vi "Trainging_Program_redesign_1세부통합.vi"() -> ()   [LabVIEW 2014]
uses:
  <vilib>/DAQmx/create/channels.llb/DAQmx Create Channel (AI-Voltage-Basic).vi
  <vilib>/DAQmx/configure/timing.llb/DAQmx Timing (Sample Clock).vi
  <vilib>/DAQmx/read.llb/DAQmx Read (Analog 1D Wfm NChan NSamp).vi
  <vilib>/Utility/file.llb/Write To Spreadsheet File (I64).vi
  <vilib>/Utility/file.llb/Write To Spreadsheet File (DBL).vi
  NeuroSky_Dll_Call/Debug/NeuroSky_Dll_Call.dll
panel:
  out "큐사인":bool
  out "실험종료":bool=TRUE
  out "icon_온도":bool
  out "icon_자판":bool
  out "icon_침대":bool
  out "icon_기계":bool
  out "icon_응급":bool=TRUE
  out "icon_용변":bool
  out "error out":errorcluster={"status"=TRUE, "code"=10, "source"="Create Folder in Trainging_Set_For_ LDA_Matrix_RSVP.vi<APPEND>\nC:\\Emotion_Research\\_Training_Test(LDA)\\2014-08-30"}
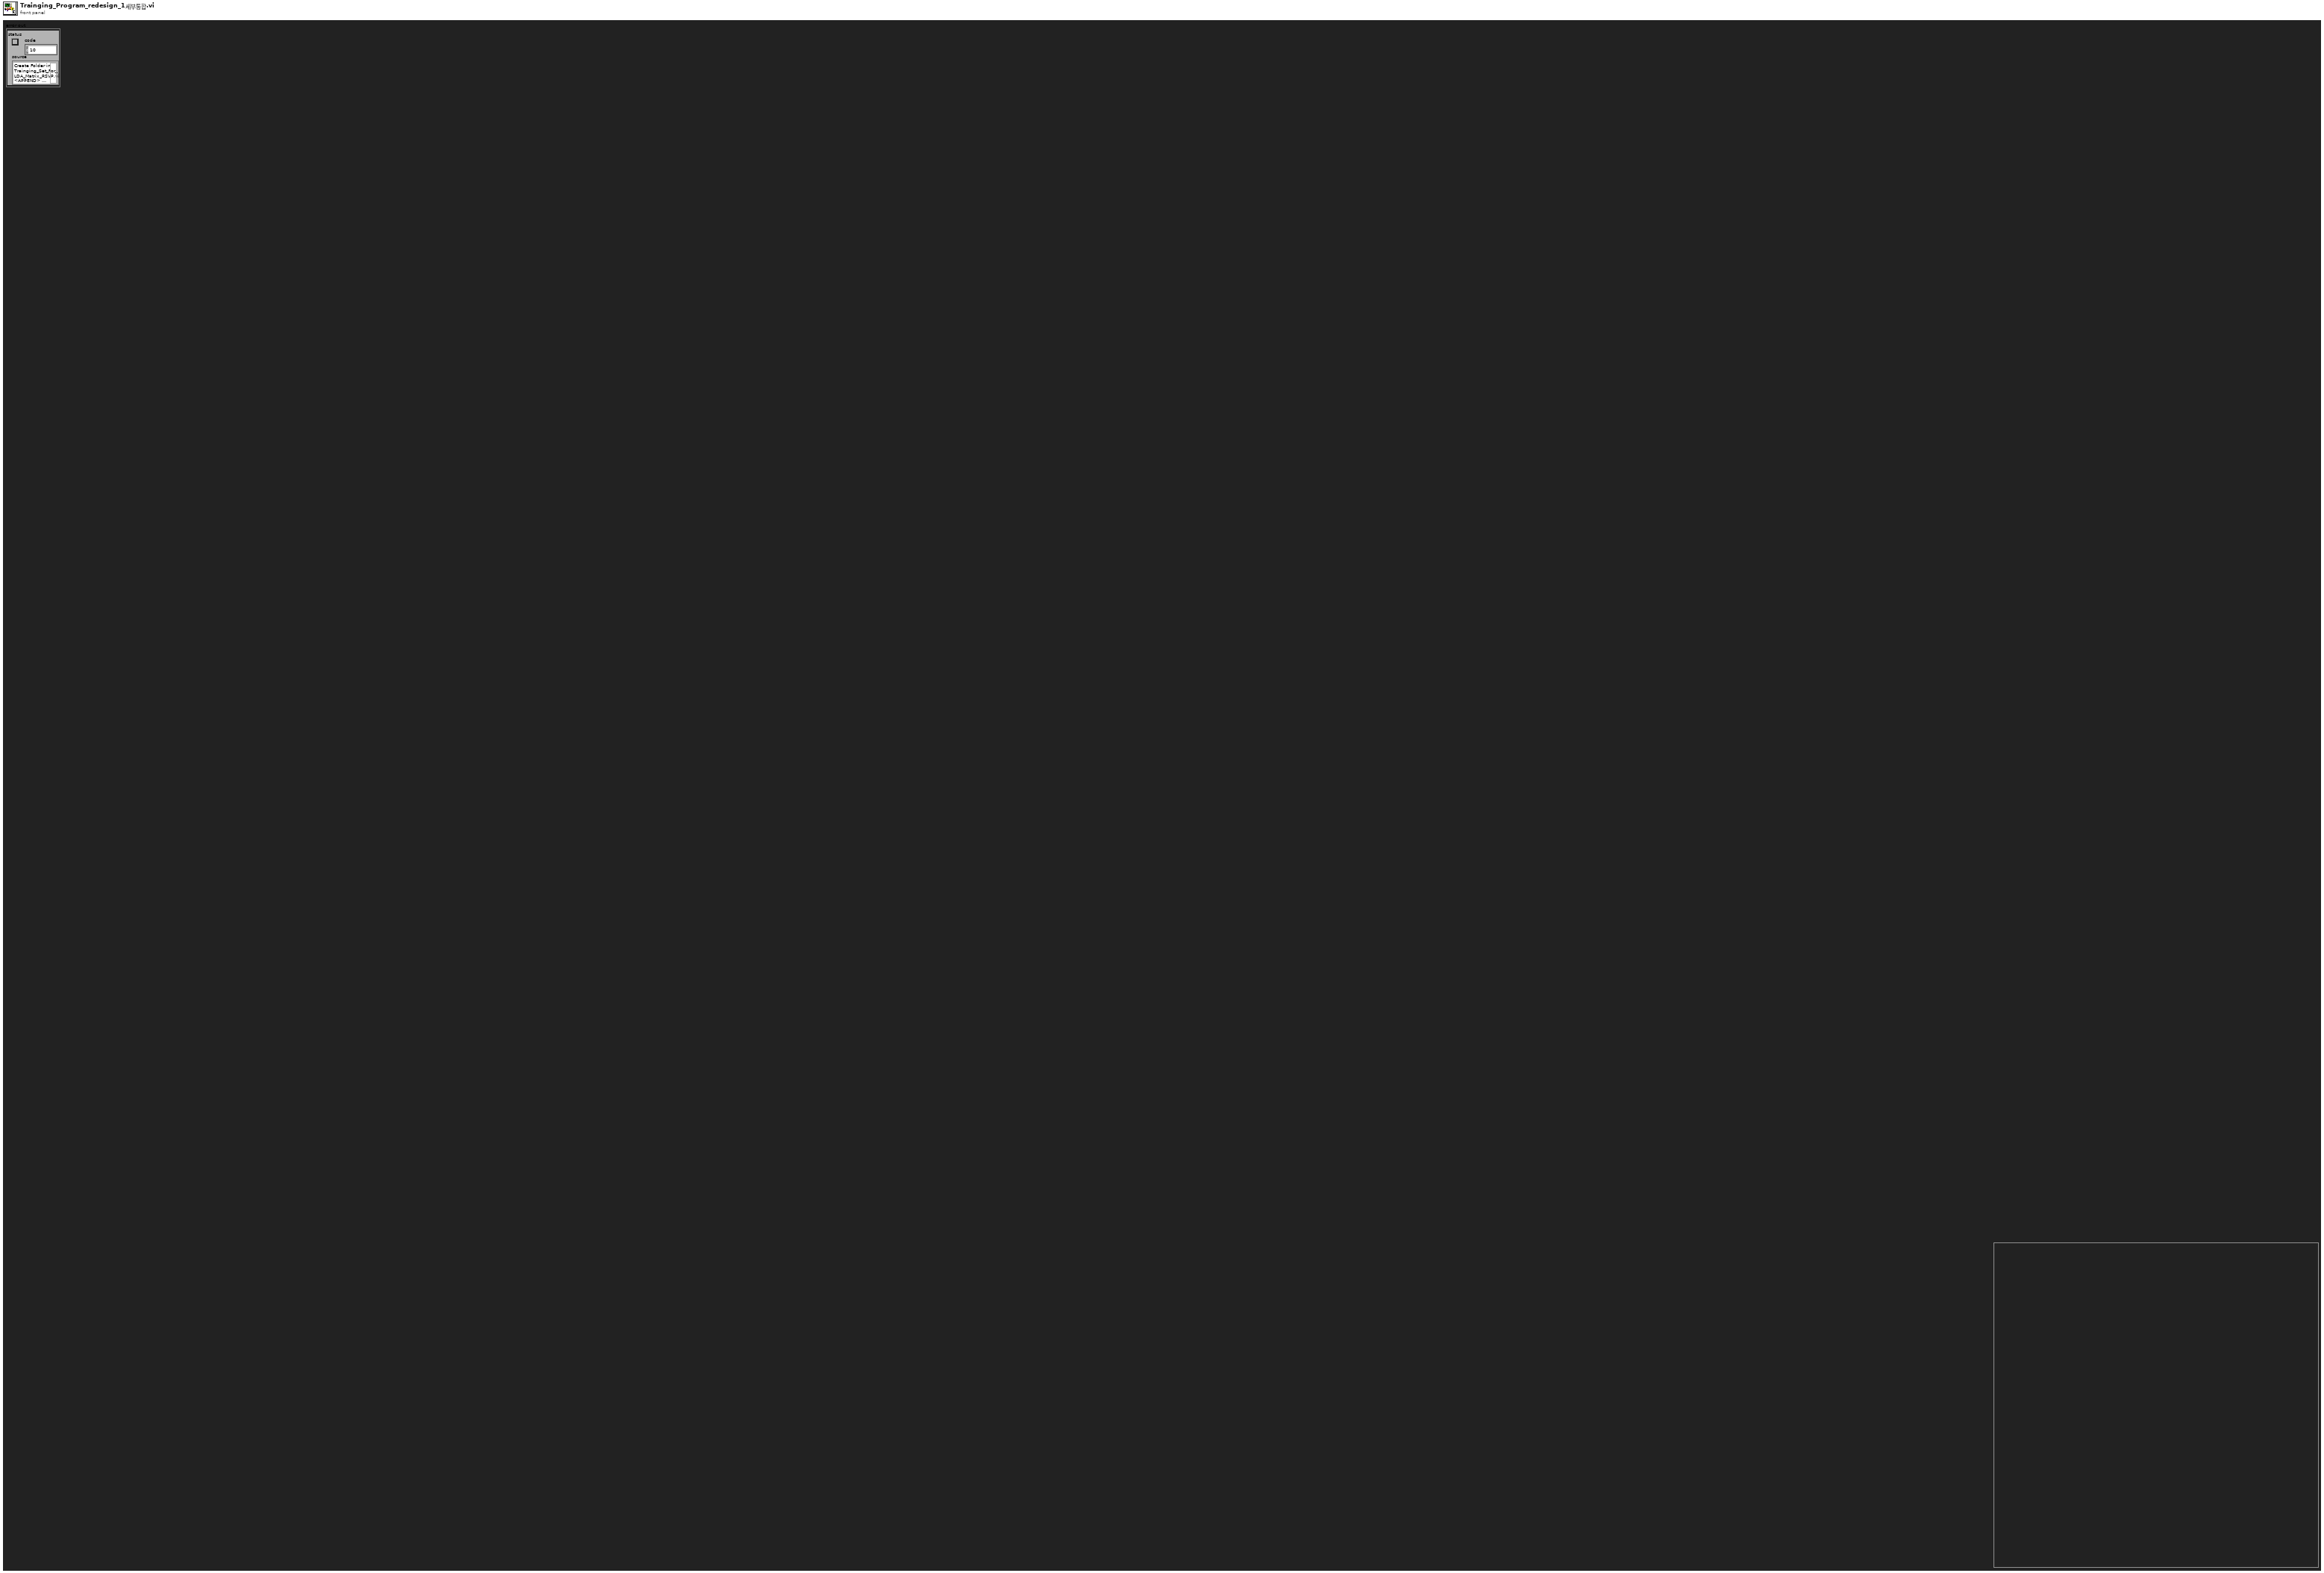
[diagram p1: front panel]
types:
  T1 = typedef "NI_Matrix.lvlib/RealMatrix.ctl" = dbl[][]
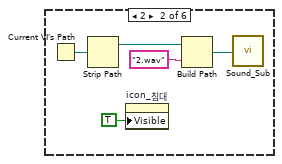
[diagram p2: hidden frame]
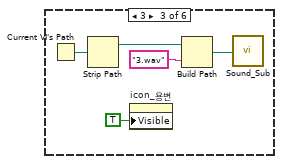
[diagram p3: hidden frame]
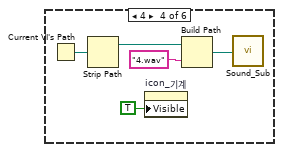
[diagram p4: hidden frame]
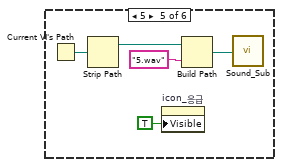
[diagram p5: hidden frame]
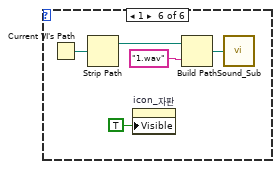
[diagram p6: hidden frame]
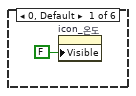
[diagram p7: hidden frame]
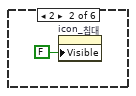
[diagram p8: hidden frame]
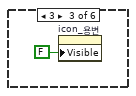
[diagram p9: hidden frame]
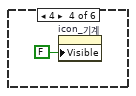
[diagram p10: hidden frame]
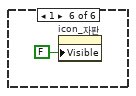
[diagram p11: hidden frame]
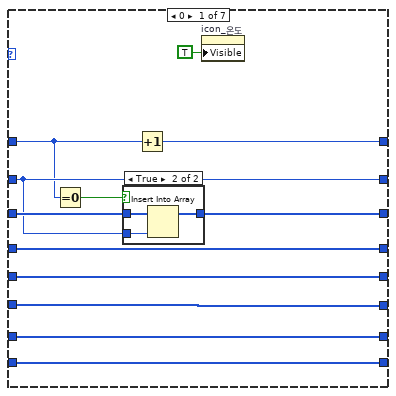
[diagram p12: hidden frame]
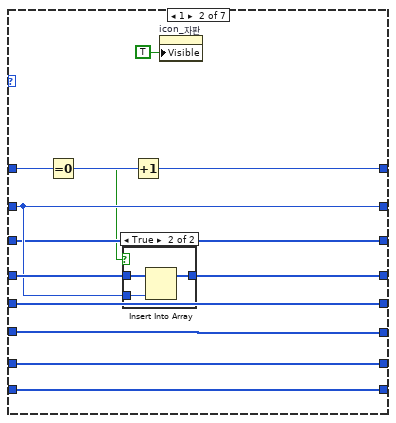
[diagram p14: hidden frame]
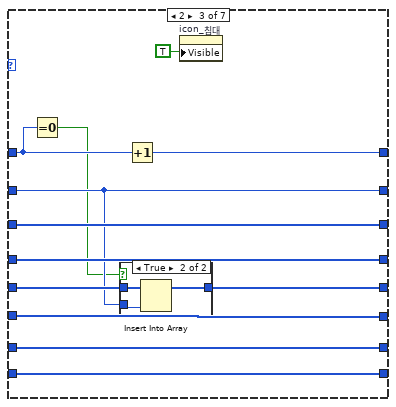
[diagram p16: hidden frame]
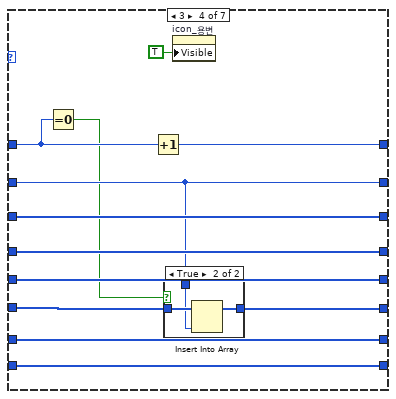
[diagram p18: hidden frame]
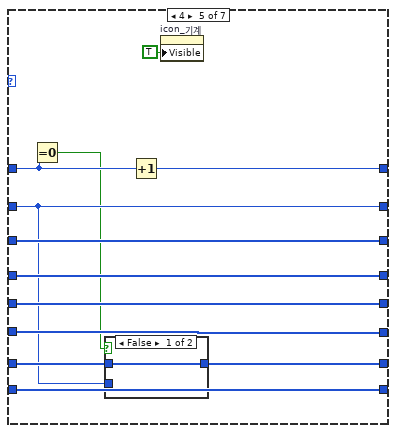
[diagram p20: hidden frame]
diagram:
  w8 = 500 ("Position:Left")
  w1 = FALSE ("Visible")
  # "0 = 온도\n1 = 자판\n2 = 침대\n3 = 용변 \n4 = 기계 \n5 = 응급"
  n1 = property on="icon_기계" class="Bool (strict)"("Left"=w8, "Top"=w8) -> ()  [unwired: 2 in, 2 out]
  n2 = property on="icon_자판" class="Bool (strict)"("Left"=w8, "Top"=w8) -> ()  [unwired: 2 in, 2 out]
  n3 = property on="icon_침대" class="Bool (strict)"("Left"=w8, "Top"=w8) -> ()  [unwired: 2 in, 2 out]
  n4 = property on="icon_응급" class="Bool (strict)"("Left"=w8, "Top"=w8) -> ()  [unwired: 2 in, 2 out]
  n5 = property on="icon_온도" class="Bool (strict)"("Left"=w8, "Top"=w8) -> ()  [unwired: 2 in, 2 out]
  n6 = property on="icon_용변" class="Bool (strict)"("Left"=w8, "Top"=w8) -> ()  [unwired: 2 in, 2 out]
  n7 = property on="실험종료" class="Bool (strict)"("Left"=200 ("Position:Left"), "Top"=600 ("Position:Top")) -> ()  [unwired: 2 in, 2 out]
  n8 = property on="큐사인" class="Bool (strict)"("Left"=w8, "Top"=w8) -> ()  [unwired: 2 in, 2 out]
  n9 = property on="큐사인" class="Bool (strict)"("Visible"=w1) -> ()  [unwired: 2 in, 2 out]
  n10 = property on="실험종료" class="Bool (strict)"("Visible"=w1) -> ()  [unwired: 2 in, 2 out]
  n11 = property on="icon_기계" class="Bool (strict)"("Visible"=w1) -> ()  [unwired: 2 in, 2 out]
  n12 = property on="icon_온도" class="Bool (strict)"("Visible"=w1) -> ()  [unwired: 2 in, 2 out]
  n13 = property on="icon_자판" class="Bool (strict)"("Visible"=w1) -> ()  [unwired: 2 in, 2 out]
  n14 = property on="icon_침대" class="Bool (strict)"("Visible"=w1) -> ()  [unwired: 2 in, 2 out]
  n15 = property on="icon_응급" class="Bool (strict)"("Visible"=w1) -> ()  [unwired: 2 in, 2 out]
  n16 = property on="icon_용변" class="Bool (strict)"("Visible"=w1) -> ()  [unwired: 2 in, 2 out]
  n17 = flat-sequence {
    tunnel: [w32] -> w31
    tunnel: w31 -> [w46]
    tunnel: [w46] -> w30
    tunnel: [w45] -> w29
    tunnel: w30 -> [w58]
    tunnel: w29 -> [w54]
    tunnel: [w58] -> w28
    tunnel: [w48] -> w27
    tunnel: [w53] -> w26
    tunnel: [w52] -> w25
    tunnel: w28 -> [w357]
    tunnel: w27 -> [w354]
    tunnel: w26 -> [w355]
    tunnel: w25 -> [w356]
    tunnel: [w357] -> w24
    tunnel: [w354] -> w23
    tunnel: [w355] -> w22
    tunnel: [w356] -> w21
    tunnel: w24 -> [w375]
    tunnel: w23 -> [w379]
    tunnel: w22 -> [w387]
    tunnel: w21 -> [w386]
    tunnel: [w374] -> w20
    tunnel: [w373] -> w19
    tunnel: [w375] -> w18
    tunnel: [w374] -> w6
    tunnel: [w373] -> w5
    tunnel: w20 -> [w404]
    tunnel: w19 -> [w414]
    tunnel: w18 -> [w399]
    tunnel: [w399] -> w17
    tunnel: w6 -> [w405]
    tunnel: w5 -> [w403]
    tunnel: [w405] -> w4
    tunnel: [w403] -> w3
    tunnel: w17 -> [w426]
    tunnel: w4 -> [w437]
    tunnel: w3 -> [w436]
    frame #0 {
      n18 = Get Date/Time In Seconds() -> (seconds since 1Jan1904=w37:timestamp)
      n19 = global read "Control_Panel_정리.vi" "피험자 이름"() -> (w33:string)
      n20 = Get Date/Time String(seconds (now)=w37) -> (date string=w36:string)  [unwired: 2 in, 1 out]
      n21 = Concatenate Strings("Emotion_Research\\" ("string"), w33, "_Training_Test(LDA)\\" ("문자열")) -> (w41:string)
      n22 = Concatenate Strings(w41, w36) -> (w39:string)
      n23 = Build Path(base path=path "C:/" ("path"), name or relative path=w39) -> (appended path=w38:path)
      n24 = Create Folder(path (use dialog)=w38) -> (created path=w32:path, error out=→"error out":errorcluster)  [unwired: 2 in, 1 out]
    }
    frame #1 {
      n25 = while {
        stop <- w47 stop-if-true
        n26 = global read "Control_Panel_정리.vi" "Start"() -> (w47:bool)
      }
      n27 = global read "Control_Panel_정리.vi" "Experimentation_num"() -> (w44:i32)
      n28 = global read "Control_Panel_정리.vi" "Random_num"() -> (w43:i32)
      n29 = call "Random2.vi"("Random_num"=w43, "전체횟수"=w44) -> ("배열"=w45:i32[])
    }
    frame #2 {
      n30 = while {
        tunnel: w54 -> [w99]
        shift-right: [w94] -> _
        shift-left: 0 ("y") -> [w95]
        shift-right: [w93] -> w52
        shift-left: i32[] [] ("subarray") -> [w82]
        shift-right: [w91] -> w48
        shift-left: dbl[][] [] -> [w92]
        shift-right: [w84] -> w53
        shift-left: i32[][] [] -> [w81]
        i -> [w90]
        stop <- w89 stop-if-true
        # "현재타겟에 해당하는 \nflash order 만 가져옴"
        n31 = flat-sequence {
          tunnel: [w103] -> w75
          tunnel: w99 -> [w105]
          tunnel: w90 -> [w104]
          tunnel: [w106] -> w73
          tunnel: w95 -> [w106]
          tunnel: [w100] -> w71
          tunnel: w75 -> [w139]
          tunnel: [w139] -> w74
          tunnel: w73 -> [w138]
          tunnel: [w138] -> w72
          tunnel: w71 -> [w137]
          tunnel: [w137] -> w70
          tunnel: w74 -> [w149]
          tunnel: [w149] -> w78
          tunnel: w72 -> [w148]
          tunnel: [w148] -> w77
          tunnel: w70 -> [w147]
          tunnel: [w147] -> w76
          tunnel: w78 -> [w153]
          tunnel: [w153] -> w69
          tunnel: w77 -> [w152]
          tunnel: [w152] -> w67
          tunnel: w76 -> [w151]
          tunnel: [w151] -> w65
          tunnel: w69 -> [w157]
          tunnel: [w157] -> w68
          tunnel: w67 -> [w156]
          tunnel: [w156] -> w66
          tunnel: w65 -> [w155]
          tunnel: [w155] -> w64
          tunnel: [w195] -> w63
          tunnel: [w194] -> w62
          tunnel: [w193] -> w61
          tunnel: [w192] -> w60
          tunnel: w64 -> [w195]
          tunnel: w66 -> [w188]
          tunnel: w68 -> [w191]
          tunnel: [w350] -> w59
          tunnel: [w351] -> w94
          tunnel: [w352] -> w87
          tunnel: [w353] -> w85
          tunnel: w63 -> [w353]
          tunnel: w62 -> [w352]
          tunnel: w61 -> [w351]
          tunnel: w60 -> [w350]
          frame #0 {
            # "타겟 순서"
            # "결과로 만들어지는 배열은 일차원배열로\n출력되면 랜덤 숫자는 0부터 시작함"
            n32 = global read "Control_Panel_정리.vi" "Random_num"() -> (w101:i32)
            n33 = global read "Control_Panel_정리.vi" "Flash_Repeat"() -> (w102:i32)
            n34 = Index Array(array=w105, index=w104) -> (element=w100:i32)
            n35 = case shown="0, Default" w100 {
              frame 0, Default {
                n36 = Current VI's Path() -> (path=w109:path)
                n37 = Strip Path(path=w109) -> (stripped path=w110:path)  [unwired: 1 out]
                n38 = property on="icon_온도" class="Bool (strict)"("Visible"=TRUE) -> ()  [unwired: 2 in, 2 out]
                n39 = Build Path(base path=w110, name or relative path="0.wav" ("이름 또는 상대 경로")) -> (appended path=w108:path)
                n40 = call "Sound_Sub.vi"("path"=w108) -> ()
              }
              frame 2 {
                n41 = Current VI's Path() -> (path=w113:path)
                n42 = Strip Path(path=w113) -> (stripped path=w114:path)  [unwired: 1 out]
                n43 = property on="icon_침대" class="Bool (strict)"("Visible"=TRUE) -> ()  [unwired: 2 in, 2 out]
                n44 = Build Path(base path=w114, name or relative path="2.wav" ("이름 또는 상대 경로")) -> (appended path=w116:path)
                n45 = call "Sound_Sub.vi"("path"=w116) -> ()
              }
              frame 3 {
                n46 = Current VI's Path() -> (path=w118:path)
                n47 = Strip Path(path=w118) -> (stripped path=w119:path)  [unwired: 1 out]
                n48 = property on="icon_용변" class="Bool (strict)"("Visible"=TRUE) -> ()  [unwired: 2 in, 2 out]
                n49 = Build Path(base path=w119, name or relative path="3.wav" ("이름 또는 상대 경로")) -> (appended path=w121:path)
                n50 = call "Sound_Sub.vi"("path"=w121) -> ()
              }
              frame 4 {
                n51 = Current VI's Path() -> (path=w123:path)
                n52 = Strip Path(path=w123) -> (stripped path=w124:path)  [unwired: 1 out]
                n53 = property on="icon_기계" class="Bool (strict)"("Visible"=TRUE) -> ()  [unwired: 2 in, 2 out]
                n54 = Build Path(base path=w124, name or relative path="4.wav" ("이름 또는 상대 경로")) -> (appended path=w126:path)
                n55 = call "Sound_Sub.vi"("path"=w126) -> ()
              }
              frame 5 {
                n56 = Current VI's Path() -> (path=w128:path)
                n57 = Strip Path(path=w128) -> (stripped path=w129:path)  [unwired: 1 out]
                n58 = property on="icon_응급" class="Bool (strict)"("Visible"=TRUE) -> ()  [unwired: 2 in, 2 out]
                n59 = Build Path(base path=w129, name or relative path="5.wav" ("이름 또는 상대 경로")) -> (appended path=w131:path)
                n60 = call "Sound_Sub.vi"("path"=w131) -> ()
              }
              frame 1 {
                n61 = Current VI's Path() -> (path=w134:path)
                n62 = Strip Path(path=w134) -> (stripped path=w135:path)  [unwired: 1 out]
                n63 = property on="icon_자판" class="Bool (strict)"("Visible"=TRUE) -> ()  [unwired: 2 in, 2 out]
                n64 = Build Path(base path=w135, name or relative path="1.wav" ("이름 또는 상대 경로")) -> (appended path=w133:path)
                n65 = call "Sound_Sub.vi"("path"=w133) -> ()
              }
            }
            n66 = call "Random2.vi"("Random_num"=w101, "전체횟수"=w102) -> ("배열"=w103:i32[])
          }
          frame #1 {
            n67 = case shown="5" w137 {
              frame 0, Default {
                n68 = property on="icon_온도" class="Bool (strict)"("Visible"=FALSE) -> ()  [unwired: 2 in, 2 out]
              }
              frame 2 {
                n69 = property on="icon_침대" class="Bool (strict)"("Visible"=FALSE) -> ()  [unwired: 2 in, 2 out]
              }
              frame 3 {
                n70 = property on="icon_용변" class="Bool (strict)"("Visible"=FALSE) -> ()  [unwired: 2 in, 2 out]
              }
              frame 4 {
                n71 = property on="icon_기계" class="Bool (strict)"("Visible"=FALSE) -> ()  [unwired: 2 in, 2 out]
              }
              frame 5 {
                n72 = property on="icon_응급" class="Bool (strict)"("Visible"=FALSE) -> ()  [unwired: 2 in, 2 out]
              }
              frame 1 {
                n73 = property on="icon_자판" class="Bool (strict)"("Visible"=FALSE) -> ()  [unwired: 2 in, 2 out]
              }
            }
          }
          frame #2 {
            n74 = property on="큐사인" class="Bool (strict)"("Visible"=TRUE) -> ()  [unwired: 2 in, 2 out]
          }
          frame #3 {
            # "2초간 큐사인을 보여줌"
            n75 = Wait (ms)(milliseconds to wait=u32 2000) -> ()  [unwired: 1 out]
          }
          frame #4 {
            n76 = property on="큐사인" class="Bool (strict)"("Visible"=FALSE) -> ()  [unwired: 2 in, 2 out]
          }
          frame #5 {
            w185 = i32[] []
            # "이 프로그램 실행시\nRate = 512Hz\nFrame Length = 40\n으로 세팅하여서 시작하여아함"
            # "random_repeat * random_num"
            n77 = global read "Control_Panel_정리.vi" "Frame Length"() -> (w161:i32)
            n78 = global read "Control_Panel_정리.vi" "sample mode"() -> (w164:i32)
            n79 = global read "Control_Panel_정리.vi" "rate"() -> (w163:dbl)
            n80 = global read "Control_Panel_정리.vi" "input terminal configuration"() -> (w169:i32)
            n81 = global read "Control_Panel_정리.vi" "physical channels"() -> (w166:tag)
            n82 = global read "Control_Panel_정리.vi" "Frame Length"() -> (w160:i32)
            n83 = global read "Control_Panel_정리.vi" "rate"() -> (w159:dbl)
            n84 = call-poly <vilib>:"DAQmx Create Virtual Channel.vi"("maximum value"=10.0, "minimum value"=-10.0, "input terminal configuration"=w169, "physical channels"=w166) -> ("task out"=w165:refnum<k21>, "error out"=w177:errorcluster)  [unwired: 10 in]
            n85 = Divide(x=w160, y=w159) -> (x/y=w158:dbl)
            n86 = call-poly <vilib>:"DAQmx Timing.vi"("task/channels in"=w165, "sample mode"=w164, "samples per channel"=w161, "rate"=w163, "error in"=w177) -> ("task out"=w162:refnum<k21>, "error out"=w178:errorcluster)  [unwired: 9 in]
            n87 = call <vilib>:"DAQmx Start Task.vi"("task/channels in"=w162, "error in"=w178) -> ("task out"=w175:refnum<k21>, "error out"=w176:errorcluster)  [unwired: 12 in]
            n88 = while {
              tunnel: w191 -> [w241]
              shift-right: [w203] -> w192
              shift-left: dbl[][] [] -> [w202]
              shift-right: [w240] -> w179
              shift-left: w185 -> [w239]
              shift-right: [w237] -> w180
              shift-left: w185 -> [w238]
              shift-right: [w235] -> w181
              shift-left: w185 -> [w236]
              shift-right: [w233] -> w182
              shift-left: w185 -> [w234]
              shift-right: [w231] -> w183
              shift-left: w185 -> [w232]
              shift-right: [w230] -> w184
              shift-left: w185 -> [w222]
              shift-right: [w228] -> w193
              shift-left: w188 -> [w229]
              shift-right: [w227] -> _
              shift-left: 0 -> [w225]
              shift-right: [w223] -> _
              shift-left: 0 ("y") -> [w224]
              tunnel: w176 -> [w205]
              tunnel: w175 -> [w206]
              tunnel: [w200] -> w171
              tunnel: [w199] -> w170
              tunnel: w161 -> [w198]
              tunnel: w158 -> [w196]
              i -> [w226]
              stop <- w207 stop-if-true
              # "ITR =  ~240ms"
              # "0 = 온도\n1 = 자판\n2 = 침대\n3 = 용변 \n4 = 기계 \n5 = 응급"
              n89 = Round Toward -Infinity(1:w196) -> (0:w197:dbl)
              n90 = global read "Control_Panel_정리.vi" "Random_num"() -> (w209:i32)
              n91 = global read "Control_Panel_정리.vi" "Flash_Repeat"() -> (w210:i32)
              n92 = Increment(x=w226) -> (x+1=w212:i32)
              n93 = call-poly <vilib>:"DAQmx Read.vi"("task/channels in"=w206, "number of samples per channel"=w198, "error in"=w205) -> ("task out"=w200:refnum<k21>, "data"=w204:waveform(dbl)[], "error out"=w199:errorcluster)  [unwired: 10 in]
              n94 = Quotient & Remainder(x=w212, y=3) -> (x-y*floor(x/y)=w217:i32)  [unwired: 1 out]
              n95 = Equal To 0?(x=w217) -> (x = 0?=w215:bool)
              n96 = Multiply(x=w210, y=w209) -> (x*y=w208:i32)
              n97 = Add(x=w197, y=w208) -> (x+y=w221:dbl)
              n98 = call "다이나믹 데이터로부터 변환"("Dynamic Data Type"=w204) -> ("Array"=w201:dbl[][])  [unwired: 3 in]
              n99 = Greater Or Equal?(x=w225, y=w208) -> (x >= y?=w214:bool)
              n100 = Increment(x=w225) -> (x+1=w216:i32)
              n101 = Increment(x=w229) -> (x+1=w219:i32)
              n102 = Equal?(x=w225, y=w221) -> (x = y?=w207:bool)
              n103 = Build Array (concatenate)(w202, w201) -> (w203:dbl[][])
              n104 = Index Array(array=w241, index=w225) -> (element=w211:i32)
              n105 = Or(x=w215, y=w214) -> (x .or. y?=w213:bool)
              n106 = Select(t=w216, s=w215, f=w225) -> (s? t:f=w227:i32)
              n107 = Select(t=w209, s=w213, f=w211) -> (s? t:f=w220:i32)
              n108 = case shown="6, Default" w220 {
                tunnel: w219 -> [w247 w263 w278 w294 w310 w327 w342]
                tunnel: [w252 w260 w285 w301 w317 w333 w348] -> w240
                tunnel: w239 -> [w253 w260 w285 w301 w317 w333 w348]
                tunnel: w238 -> [w251 w269 w282 w298 w314 w331 w347]
                tunnel: [w251 w268 w282 w298 w314 w331 w347] -> w237
                tunnel: w236 -> [w250 w267 w284 w297 w313 w330 w346]
                tunnel: [w250 w267 w283 w297 w313 w330 w346] -> w235
                tunnel: w234 -> [w249 w266 w281 w300 w312 w329 w345]
                tunnel: [w249 w266 w281 w299 w312 w329 w345] -> w233
                tunnel: w232 -> [w248 w265 w280 w296 w316 w328 w344]
                tunnel: [w248 w265 w280 w296 w315 w328 w344] -> w231
                tunnel: w222 -> [w244 w264 w279 w295 w311 w332 w343]
                tunnel: [w244 w264 w279 w295 w311 w324 w343] -> w230
                tunnel: [w247 w263 w278 w294 w310 w327 w342] -> w228
                tunnel: w224 -> [w246 w262 w277 w292 w309 w325 _]
                tunnel: [w245 w261 w276 w293 w308 w326 0] -> w223
                frame 0 {
                  n109 = Equal To 0?(x=w246) -> (x = 0?=w242:bool)
                  n110 = case shown="True" w242 {
                    tunnel: w253 -> [w254 w257]
                    tunnel: [w254 w256] -> w252
                    tunnel: w247 -> [_ w255]
                    frame False {
                    }
                    frame True {
                      n111 = Insert Into Array(array=w257, new element=w255) -> (w256:i32[])  [unwired: 1 in]
                    }
                  }
                  n112 = Increment(x=w246) -> (x+1=w245:i32)
                  n113 = property on="icon_온도" class="Bool (strict)"("Visible"=TRUE) -> ()  [unwired: 2 in, 2 out]
                }
                frame 1 {
                  n114 = Equal To 0?(x=w262) -> (x = 0?=w258:bool)
                  n115 = case shown="True" w258 {
                    tunnel: w269 -> [w270 w273]
                    tunnel: [w270 w272] -> w268
                    tunnel: w263 -> [_ w271]
                    frame False {
                    }
                    frame True {
                      n116 = Insert Into Array(array=w273, new element=w271) -> (w272:i32[])  [unwired: 1 in]
                    }
                  }
                  n117 = Increment(x=w262) -> (x+1=w261:i32)
                  n118 = property on="icon_자판" class="Bool (strict)"("Visible"=TRUE) -> ()  [unwired: 2 in, 2 out]
                }
                frame 2 {
                  n119 = Equal To 0?(x=w277) -> (x = 0?=w274:bool)
                  n120 = case shown="True" w274 {
                    tunnel: w284 -> [w286 w289]
                    tunnel: [w286 w288] -> w283
                    tunnel: w278 -> [_ w287]
                    frame False {
                    }
                    frame True {
                      n121 = Insert Into Array(array=w289, new element=w287) -> (w288:i32[])  [unwired: 1 in]
                    }
                  }
                  n122 = Increment(x=w277) -> (x+1=w276:i32)
                  n123 = property on="icon_침대" class="Bool (strict)"("Visible"=TRUE) -> ()  [unwired: 2 in, 2 out]
                }
                frame 3 {
                  n124 = Equal To 0?(x=w292) -> (x = 0?=w290:bool)
                  n125 = Increment(x=w292) -> (x+1=w293:i32)
                  n126 = case shown="True" w290 {
                    tunnel: w300 -> [w302 w305]
                    tunnel: [w302 w304] -> w299
                    tunnel: w294 -> [_ w303]
                    frame False {
                    }
                    frame True {
                      n127 = Insert Into Array(array=w305, new element=w303) -> (w304:i32[])  [unwired: 1 in]
                    }
                  }
                  n128 = property on="icon_용변" class="Bool (strict)"("Visible"=TRUE) -> ()  [unwired: 2 in, 2 out]
                }
                frame 4 {
                  n129 = Equal To 0?(x=w309) -> (x = 0?=w306:bool)
                  n130 = case shown="False" w306 {
                    tunnel: w316 -> [w318 w321]
                    tunnel: [w318 w320] -> w315
                    tunnel: w310 -> [_ w319]
                    frame False {
                    }
                    frame True {
                      n131 = Insert Into Array(array=w321, new element=w319) -> (w320:i32[])  [unwired: 1 in]
                    }
                  }
                  n132 = Increment(x=w309) -> (x+1=w308:i32)
                  n133 = property on="icon_기계" class="Bool (strict)"("Visible"=TRUE) -> ()  [unwired: 2 in, 2 out]
                }
                frame 5 {
                  n134 = Equal To 0?(x=w325) -> (x = 0?=w322:bool)
                  n135 = Increment(x=w325) -> (x+1=w326:i32)
                  n136 = property on="icon_응급" class="Bool (strict)"("Visible"=TRUE) -> ()  [unwired: 2 in, 2 out]
                  n137 = case shown="True" w322 {
                    tunnel: w332 -> [w334 w337]
                    tunnel: [w334 w336] -> w324
                    tunnel: w327 -> [_ w335]
                    frame False {
                    }
                    frame True {
                      n138 = Insert Into Array(array=w337, new element=w335) -> (w336:i32[])  [unwired: 1 in]
                    }
                  }
                }
                frame 6, Default {
                  w339 = FALSE ("Visible")
                  w338 = FALSE ("Visible")
                  w340 = FALSE ("Visible")
                  n139 = property on="icon_응급" class="Bool (strict)"("Visible"=w340) -> ()  [unwired: 2 in, 2 out]
                  n140 = property on="icon_용변" class="Bool (strict)"("Visible"=w340) -> ()  [unwired: 2 in, 2 out]
                  n141 = property on="icon_기계" class="Bool (strict)"("Visible"=w338) -> ()  [unwired: 2 in, 2 out]
                  n142 = property on="icon_온도" class="Bool (strict)"("Visible"=w338) -> ()  [unwired: 2 in, 2 out]
                  n143 = property on="icon_침대" class="Bool (strict)"("Visible"=w339) -> ()  [unwired: 2 in, 2 out]
                  n144 = property on="icon_자판" class="Bool (strict)"("Visible"=w339) -> ()  [unwired: 2 in, 2 out]
                }
              }
            }
            n145 = call <vilib>:"DAQmx Stop Task.vi"("task/channels in"=w171, "error in"=w170) -> ("task out"=w172:refnum<k21>, "error out"=w173:errorcluster)  [unwired: 12 in]
            n146 = call <vilib>:"DAQmx Clear Task.vi"("task in"=w172, "error in"=w173) -> ("error out"=w174:errorcluster)  [unwired: 13 in]
            n147 = call <vilib>:"Simple Error Handler.vi"("error in (no error)"=w174) -> ()  [unwired: 4 in, 5 out]
            n148 = Build Array(w179, w180, w181, w182, w183, w184) -> (w189:i32[][])
            n149 = Transpose 2D Array(2D array=w189) -> (transposed array=w194:i32[][])
          }
          frame #6 {
            w349 = FALSE ("Visible")
            n150 = property on="icon_자판" class="Bool (strict)"("Visible"=w349) -> ()  [unwired: 2 in, 2 out]
            n151 = property on="icon_기계" class="Bool (strict)"("Visible"=w349) -> ()  [unwired: 2 in, 2 out]
            n152 = property on="icon_침대" class="Bool (strict)"("Visible"=w349) -> ()  [unwired: 2 in, 2 out]
            n153 = property on="icon_응급" class="Bool (strict)"("Visible"=w349) -> ()  [unwired: 2 in, 2 out]
            n154 = property on="icon_온도" class="Bool (strict)"("Visible"=w349) -> ()  [unwired: 2 in, 2 out]
            n155 = property on="icon_용변" class="Bool (strict)"("Visible"=w349) -> ()  [unwired: 2 in, 2 out]
          }
        }
        n156 = global read "Control_Panel_정리.vi" "Experimentation_num"() -> (w80:i32)
        n157 = global read "Control_Panel_정리.vi" "Random_num"() -> (w79:i32)
        n158 = Multiply(x=w80, y=w79) -> (x*y=w97:i32)
        n159 = Subtract(x=w97, y=2) -> (x-y=w98:i32)
        n160 = Greater?(x=w90, y=w98) -> (0:w89:bool)
        n161 = Index Array(array=w87, index (col)=w85) -> (element=w88:i32[])  [unwired: 1 in]
        n162 = Insert Into Array(array=w92, new element=w59) -> (w91:dbl[][])  [unwired: 2 in]
        n163 = Delete From Array(array=w87, length=1 ("길이"), index (col)=w85) -> (array with subset deleted=w86:i32[][])  [unwired: 1 in, 1 out]
        n164 = Build Array (concatenate)(w81, w86) -> (w84:i32[][])
        n165 = Insert Into Array(array=w82, new element=w88) -> (w93:i32[])  [unwired: 1 in]
      }
      n166 = global write "Control_Panel_정리.vi" "Acquisition Mode"(TRUE ("Device Control Enabled")) -> ()
      n167 = global write "Control_Panel_정리.vi" "Device Control Enabled"(FALSE ("Device Control Enabled")) -> ()
    }
    frame #3 {
      # "현재타겟에 해당하는 \nflash order 만 가져옴"
      # "target=stimulus 때의 order만 가져옴"
      n168 = flat-sequence {
        frame #0 {
          n169 = dll-call lib="PTH2uabs CUsersJaehongDesktop연구_programNeuroSky_최종본NeuroSky_Dll_CallDebugNeuroSky_Dll_Call.dll" fn="FreeConnection"() -> ()  [unwired: 4 in, 2 out]
        }
        frame #1 {
          n170 = property on="실험종료" class="Bool (strict)"("Visible"=TRUE) -> ()  [unwired: 2 in, 2 out]
        }
        frame #2 {
          n171 = global write "Control_Panel_정리.vi" "Value Achieving Status"("All Connection terminated,\nExperiment over" ("name or relative path")) -> ()
          n172 = global write "Control_Panel_정리.vi" "Acquisition Mode"(FALSE ("Device Control Enabled")) -> ()
        }
      }
      n173 = Build Path(base path=w357, name or relative path="Brain.txt") -> (appended path=w360:path)
      n174 = Build Path(base path=w357, name or relative path="Target_order.txt") -> (appended path=w363:path)
      n175 = call-poly <vilib>:"Write To Spreadsheet File.vi"("transpose? (no:F)"=TRUE, "1D data"=w356, "file path (dialog if empty)"=w363) -> ()  [unwired: 5 in, 1 out]
      n176 = Build Path(base path=w357, name or relative path="Nontarget_order.txt") -> (appended path=w364:path)
      n177 = call-poly <vilib>:"Write To Spreadsheet File.vi"("format (%.3f)"="%.6f", "2D data"=w354, "file path (dialog if empty)"=w360) -> ()  [unwired: 5 in, 1 out]
      n178 = call-poly <vilib>:"Write To Spreadsheet File.vi"("transpose? (no:F)"=FALSE, "2D data"=w355, "file path (dialog if empty)"=w364) -> ()  [unwired: 5 in, 1 out]
    }
    frame #4 {
      n179 = global read "Control_Panel_정리.vi" "Experimentation_num"() -> (w390:i32)
      n180 = global read "Control_Panel_정리.vi" "Flash_Repeat"() -> (w392:i32)
      n181 = global read "Control_Panel_정리.vi" "Random_num"() -> (w391:i32)
      n182 = global write "Control_Panel_정리.vi" "Communication Stopped"(TRUE ("Device Control Enabled")) -> ()
      n183 = global read "Control_Panel_정리.vi" "Frame Length"() -> (w388:i32)
      n184 = global read "Control_Panel_정리.vi" "rate"() -> (w389:dbl)
      n185 = call "Subvi_Training_Baseline_w_range_w_weight_1세부통합.vi"("Nontarget_Flash_Order"=w387, "Target_Flash_Order"=w386, "samples per channel"=w388, "Brain_data_source"=w379, "rate"=w389, "Experimentation_num"=w390, "Random_num"=w391, "Random_Repeat"=w392) -> ("Target_ERP"=w370:dbl[][], "NonTarget"=w373:dbl[][], "Nontarget_ERP"=w371:dbl[][], "Target"=w374:dbl[][])
      n186 = Build Path(base path=w375, name or relative path="Nontarget_ERP_AVG.txt") -> (appended path=w377:path)
      n187 = Build Path(base path=w375, name or relative path="Target_ERP_AVG.txt") -> (appended path=w394:path)
      n188 = Build Path(base path=w375, name or relative path="ERP_Parameters_of_Target_prior.txt") -> (appended path=w384:path)
      n189 = Build Path(base path=w375, name or relative path="ERP_Parameters_of_NonTarget_prior.txt") -> (appended path=w381:path)
      n190 = call-poly <vilib>:"Write To Spreadsheet File.vi"("format (%.3f)"="%.6f", "2D data"=w371, "file path (dialog if empty)"=w377) -> ()  [unwired: 5 in, 1 out]
      n191 = call-poly <vilib>:"Write To Spreadsheet File.vi"("format (%.3f)"="%.6f", "2D data"=w370, "file path (dialog if empty)"=w394) -> ()  [unwired: 5 in, 1 out]
      n192 = call-poly <vilib>:"Write To Spreadsheet File.vi"("format (%.3f)"="%.6f", "2D data"=w374, "file path (dialog if empty)"=w384) -> ()  [unwired: 5 in, 1 out]
      n193 = call-poly <vilib>:"Write To Spreadsheet File.vi"("format (%.3f)"="%.6f", "2D data"=w373, "file path (dialog if empty)"=w381) -> ()  [unwired: 5 in, 1 out]
    }
    frame #5 {
      n194 = Array Size(array=w404) -> (size(s)=w417:i32[])
      n195 = Array Size(array=w414) -> (size(s)=w418:i32[])
      n196 = Index Array(array=w417) -> (element=w419:i32)  [unwired: 1 in]
      n197 = Index Array(array=w418) -> (element=w420:i32)  [unwired: 1 in]
      n198 = for {
        N: w420 -> [_]
        tunnel: [1] -> w422 mode=indexing
      }
      n199 = for {
        N: w419 -> [_]
        tunnel: [0] -> w421 mode=indexing
      }
      n200 = Build Array (concatenate)(w421, w422) -> (w413:i32[])
      n201 = Build Array (concatenate)(w404, w414) -> (w415:dbl[][])
      n202 = global read "Control_Panel_정리.vi" "EEG_Channel_Num"() -> (w396:i32)
      n203 = Insert Into Array(array=w415, index (col)=0 ("비활성화된 인덱스 (열)"), new element=w413) -> (w409:dbl[][])  [unwired: 1 in]
      n204 = call "Subvi_Training_LDA.vi"("Input_Data"=w409) -> ("A * B 2"=w407:T1, "A * B"=w408:T1)
      n205 = Initialize Array(0.090909 ("element"), w396) -> (w398:dbl[])
      n206 = Build Array (concatenate)(w408, w407) -> (w406:T1)
      n207 = Build Path(base path=w399, name or relative path="Weight_Vector_prior.txt") -> (appended path=w402:path)
      n208 = Build Path(base path=w399, name or relative path="LDA_Matrix_Value_prior.txt") -> (appended path=w411:path)
      n209 = call-poly <vilib>:"Write To Spreadsheet File.vi"("format (%.3f)"="%.6f", "1D data"=w398, "file path (dialog if empty)"=w402) -> ()  [unwired: 5 in, 1 out]
      n210 = call-poly <vilib>:"Write To Spreadsheet File.vi"("format (%.3f)"="%.6f", "2D data"=w406, "file path (dialog if empty)"=w411) -> ()  [unwired: 5 in, 1 out]
    }
    frame #6 {
      (unwired) "%.6f" ("format (%.3f)")
      # "EEG_Channel_Num과\nExperimentation_num\n조정하여 사용할것"
      # "addpath('C:\\Users\\Jaehong\\Desktop\\연구_program\\libsvm-3.18\\matlab');"
      n211 = call "SWLDA_통합버전용.vi"("premove"=0.05, "penter"=0.01, "ERP_Nontarget"=w436, "ERP_Target"=w437) -> ("in"=w425:dbl[], "LDA_matrix"=w441:T1)  [unwired: 5 in, 1 out]
      n212 = global read "Control_Panel_정리.vi" "EEG_Channel_Num"() -> (w430:i32)
      n213 = global read "Control_Panel_정리.vi" "EEG_Channel_Num"() -> (w440:i32)
      n214 = global read "Control_Panel_정리.vi" "Random_num"() -> (w439:i32)
      n215 = global read "Control_Panel_정리.vi" "Experimentation_num"() -> (w438:i32)
      n216 = Initialize Array(0.090909 ("element"), w430) -> (w432:dbl[])
      n217 = script code="%addpath to the libsvm toolbox\n\naddpath('C:\\Users\\Server\\Desktop\\NeuroSky\\RSVP_NeuroSky\\libsvm-3.18\\matlab');\n\n%read data set(training)\n\nrow_num = chan_num*4;\ncol_num = icon_num*exp_num;\n\nWeight = Weight';\nnonzeros = find(Weight, row_num);\ntarget = reshape(target', row_num, col_num);\ntarget = target.*Weight(:,ones(1,col_num));\ntarget = target(nonzeros,:);\nnontarget = reshape(nontarget', row_num, col_num);\nnontarget = nontarget.*Weight(:,ones(1,col_num));\nnontarget = nontarget(nonzeros,:);\nEEG_train = [target';nontarget']';\nlength = size(target,2);\ntrainLabel = [ones(length,1);-ones(length, 1)];\n\n% Train the SVM\n\nmodel = ...\nsvmtrain(trainLabel, [(1:col_num*2)' EEG_train'*EEG_train], '-c 1 -g 0.07 -b 1 -t 4 -q');\n\n%save model file\nsvm_savemodel(model,'C:\\WORK\\svm_model.model');" ("Script Node")("Weight"=w425, "target"=w436, "nontarget"=w437, "icon_num"=w439, "chan_num"=w440, "exp_num"=w438) -> ()  [unwired: 1 in, 1 out]
      n218 = Build Path(base path=w426, name or relative path="LDA_Matrix_Value_SWLDA.txt") -> (appended path=w444:path)
      n219 = Build Path(base path=w426, name or relative path="in_SWLDA.txt") -> (appended path=w429:path)
      n220 = Build Path(base path=w426, name or relative path="Weight_Vector_SWLDA.txt") -> (appended path=w435:path)
      n221 = call-poly <vilib>:"Write To Spreadsheet File.vi"("2D data"=w441, "file path (dialog if empty)"=w444) -> ()  [unwired: 6 in, 1 out]
      n222 = call-poly <vilib>:"Write To Spreadsheet File.vi"("format (%.3f)"="%.6f", "1D data"=w425, "file path (dialog if empty)"=w429) -> ()  [unwired: 5 in, 1 out]
      n223 = call-poly <vilib>:"Write To Spreadsheet File.vi"("format (%.3f)"="%.6f", "1D data"=w432, "file path (dialog if empty)"=w435) -> ()  [unwired: 5 in, 1 out]
    }
    frame #7 {
      n224 = global write "Control_Panel_정리.vi" "Communication Stopped"(FALSE ("Device Control Enabled")) -> ()
    }
  }
  "icon_온도" <- FALSE ("icon_전원 6")
  "icon_용변" <- FALSE ("icon_전체종료")
  "icon_자판" <- FALSE ("icon_음량업 2")
  "icon_응급" <- FALSE ("icon_채널다운")
  "icon_기계" <- FALSE ("icon_음량다")
  "icon_침대" <- FALSE ("icon_채널업")
  "실험종료" <- TRUE ("Boolean")
  "큐사인" <- FALSE ("icon_전원 7")
